vi "Init.vi"(0 "Com Port in":refnum<visa-resource-name>, 1 "error in":errorcluster caption="error out") -> (2 "COM Port out":refnum<visa-resource-name>, 3 "Device Information":T1, 4 "Init Complete":bool, 5 "error out":errorcluster)   [LabVIEW 2013]
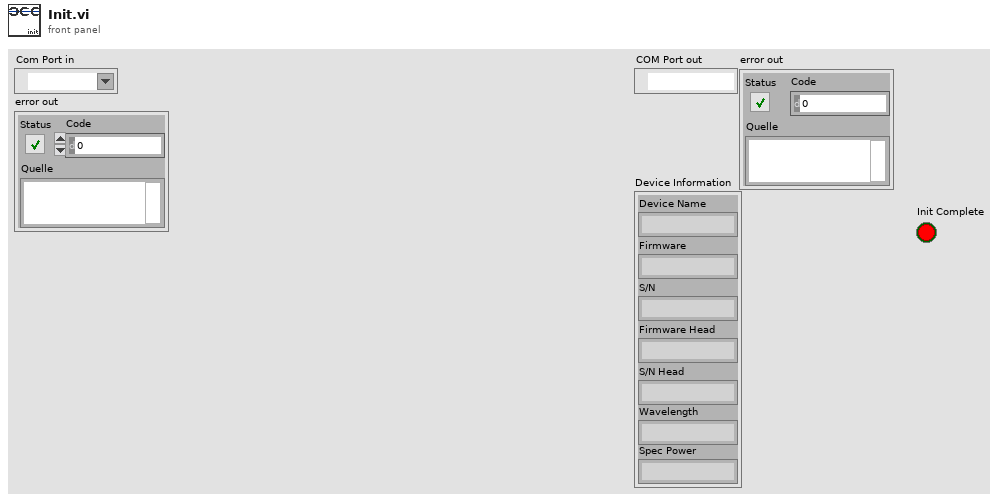
[diagram p1: front panel]
types:
  T1 = cluster{"Device Name":string, "Firmware":string, "S/N":string, "Firmware Head":string, "S/N Head":string, "Wavelength":string, "Spec Power":string}
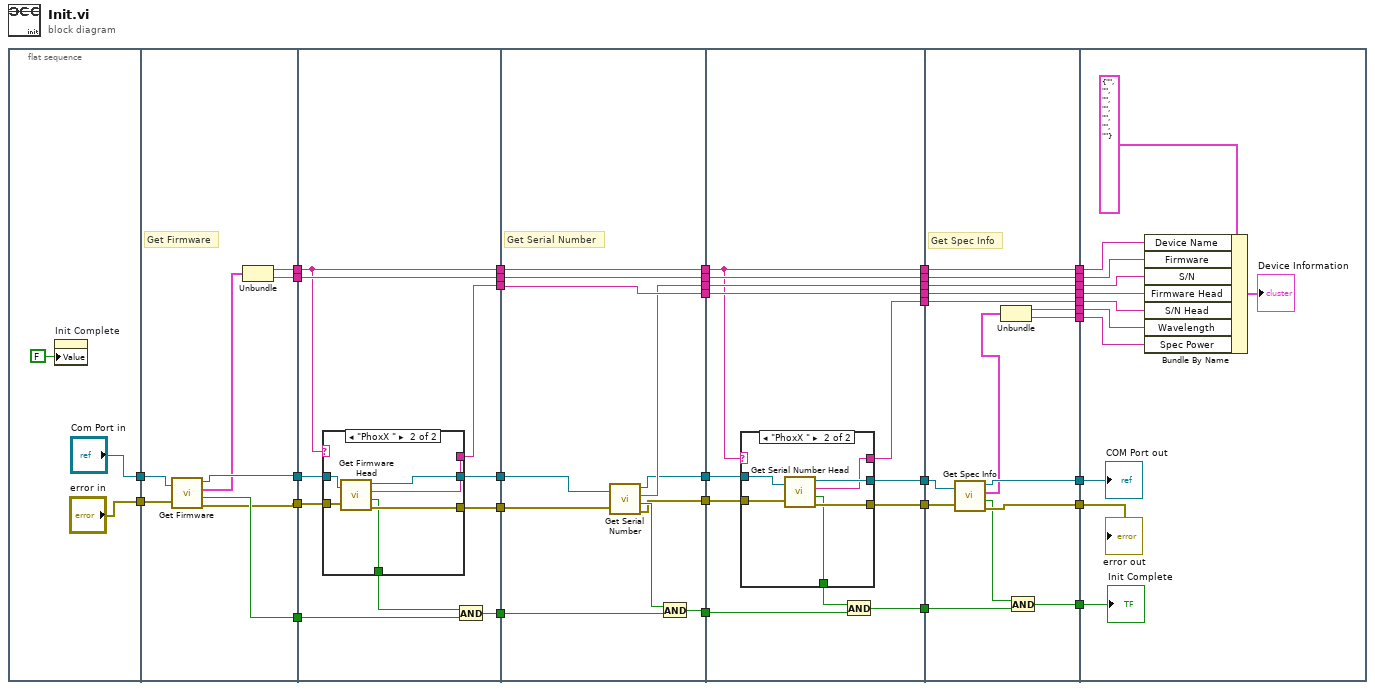
[diagram p0: block diagram]
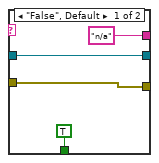
[diagram p2: hidden frame]
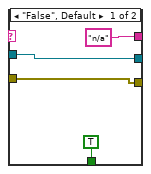
[diagram p3: hidden frame]
diagram:
  n1 = flat-sequence {
    tunnel: ["error in"] -> w38
    tunnel: ["Com Port in"] -> w37
    tunnel: w38 -> [w49]
    tunnel: [w48] -> w30
    tunnel: [w45] -> w28
    tunnel: [w43] -> w26
    tunnel: [w42] -> w24
    tunnel: w37 -> [w46]
    tunnel: [w47] -> w22
    tunnel: w30 -> [w58]
    tunnel: [w55] -> w29
    tunnel: w28 -> [w57]
    tunnel: [w56] -> w27
    tunnel: w26 -> [w50]
    tunnel: [w50] -> w25
    tunnel: w24 -> [w59]
    tunnel: [w59] -> w23
    tunnel: w22 -> [w53]
    tunnel: [w52] -> w21
    tunnel: [w51] -> w20
    tunnel: w29 -> [w75]
    tunnel: w27 -> [w74]
    tunnel: w25 -> [w76]
    tunnel: [w76] -> w36
    tunnel: w23 -> [w80]
    tunnel: [w80] -> w35
    tunnel: [w71] -> w34
    tunnel: w21 -> [w79]
    tunnel: [w78] -> w33
    tunnel: [w72] -> w32
    tunnel: w20 -> [w77]
    tunnel: [w77] -> w31
    tunnel: [w70] -> w19
    tunnel: [w87] -> w18
    tunnel: w36 -> [w81]
    tunnel: [w81] -> w16
    tunnel: w35 -> [w92]
    tunnel: [w92] -> w14
    tunnel: w34 -> [w89]
    tunnel: [w86] -> w12
    tunnel: w33 -> [w83]
    tunnel: [w82] -> w10
    tunnel: w32 -> [w91]
    tunnel: [w91] -> w8
    tunnel: w31 -> [w90]
    tunnel: [w90] -> w6
    tunnel: [w85] -> w4
    tunnel: w19 -> [w88]
    tunnel: w18 -> [w110]
    tunnel: [w109] -> w17
    tunnel: w16 -> [w117]
    tunnel: [w117] -> w15
    tunnel: w14 -> [w116]
    tunnel: [w116] -> w13
    tunnel: w12 -> [w112]
    tunnel: [w111] -> w11
    tunnel: w10 -> [w107]
    tunnel: [w106] -> w9
    tunnel: w8 -> [w115]
    tunnel: [w115] -> w7
    tunnel: w6 -> [w114]
    tunnel: [w114] -> w5
    tunnel: w4 -> [w113]
    tunnel: [w113] -> w3
    tunnel: [w104] -> w2
    tunnel: [w103] -> w1
    tunnel: w17 -> [w122]
    tunnel: w15 -> [w128]
    tunnel: w13 -> [w129]
    tunnel: w11 -> [w123]
    tunnel: w9 -> [w127]
    tunnel: w7 -> [w126]
    tunnel: w5 -> [w125]
    tunnel: w3 -> [w124]
    tunnel: w2 -> [w121]
    tunnel: w1 -> [w120]
    frame #0 {
      n2 = property on="Init Complete" class="Bool. (strikt)"("Value"=FALSE ("Init Complete")) -> ()  [unwired: 2 in, 2 out]
    }
    frame #1 {
      # "Get Firmware"
      n3 = call "Get Firmware.vi"("COM Port In"=w46, "error in"=w49) -> ("COM Port out"=w48:refnum<visa-resource-name>, "Firmware"=w44:cluster{string, "read buffer":string}, "OK"=w47:bool, "error out"=w45:errorcluster)
      n4 = Unbundle(w44) -> (w43:string, "read buffer"=w42:string)
    }
    frame #2 {
      n5 = case shown="\"PhoxX \"" w50 {
        tunnel: w58 -> [w63 w69]
        tunnel: w57 -> [w62 w65]
        tunnel: [w62 w68] -> w56
        tunnel: [w63 w67] -> w55
        tunnel: [TRUE ("OK") w64] -> w54
        tunnel: ["n/a" ("Firmware Head") w66] -> w51
        frame "False", Default {
        }
        frame "PhoxX " {
          n6 = call "Get Firmware Head.vi"("COM Port In"=w69, "error in"=w65) -> ("COM Port out"=w67:refnum<visa-resource-name>, "Firmware Head"=w66:string, "OK"=w64:bool, "error out"=w68:errorcluster)
        }
      }
      n7 = And(x=w54, y=w53) -> (x .and. y?=w52:bool)
    }
    frame #3 {
      # "Get Serial Number"
      n8 = call "Get Serial Number.vi"("COM Port in"=w75, "error in"=w74) -> ("COM Port out"=w71:refnum<visa-resource-name>, "S/N"=w72:string, "OK"=w73:bool, "error out"=w70:errorcluster)
      n9 = And(x=w73, y=w79) -> (x .and. y?=w78:bool)
    }
    frame #4 {
      n10 = case shown="\"PhoxX \"" w81 {
        tunnel: w89 -> [w96 w102]
        tunnel: w88 -> [w95 w101]
        tunnel: [w95 w100] -> w87
        tunnel: [w96 w99] -> w86
        tunnel: ["n/a" ("S/N Head") w97] -> w85
        tunnel: [TRUE ("OK") w98] -> w84
        frame "False", Default {
        }
        frame "PhoxX " {
          n11 = call "Get Serial Number Head.vi"("COM Port in"=w102, "error in"=w101) -> ("COM Port out"=w99:refnum<visa-resource-name>, "S/N Head"=w97:string, "OK"=w98:bool, "error out"=w100:errorcluster)
        }
      }
      n12 = And(x=w84, y=w83) -> (x .and. y?=w82:bool)
    }
    frame #5 {
      # "Get Spec Info"
      n13 = call "Get Spec Info.vi"("COM Port In"=w112, "error out"=w110) -> ("COM Port out"=w111:refnum<visa-resource-name>, "Spec Info"=w105:cluster{string, "read buffer":string}, "OK"=w108:bool, "error out 2"=w109:errorcluster)
      n14 = Unbundle(w105) -> (w104:string, "read buffer"=w103:string)
      n15 = And(x=w108, y=w107) -> (x .and. y?=w106:bool)
    }
    frame #6 {
      n16 = Bundle By Name(cluster=T1 {"Device Name"="", "Firmware"="", "S/N"="", "Firmware Head"="", "S/N Head"="", "Wavelength"="", "Spec Power"=""} ("Ausgangs-Cluster"), "Device Name"=w128, "Firmware"=w129, "S/N"=w126, "Firmware Head"=w125, "S/N Head"=w124, "Wavelength"=w121, "Spec Power"=w120) -> (→"Device Information":T1)
      "Init Complete" <- w127
      "COM Port out" <- w123
      "error out" <- w122
    }
  }
